vi "GetParam.vi"(8 "error in (no error)":errorcluster caption="entrée d'erreur (pas d'erreur)", 11 "Chi2_kernel.lvclass":refnum<class "Chi2_kernel.lvclass">) -> (0 "error out":errorcluster caption="sortie d'erreur", 2 "chi2_kernel":cluster{"gamma":dbl}={"gamma"=1.0}, 3 "Chi2_kernel.lvclass":refnum<class "Chi2_kernel.lvclass">)   [LabVIEW 2020, in "Chi2_kernel.lvclass"]
doc: "Get Parameters"
uses:
  Chi2_kernel.lvclass
  Chi2_kernel.lvclass/Chi2_kernel.ctl
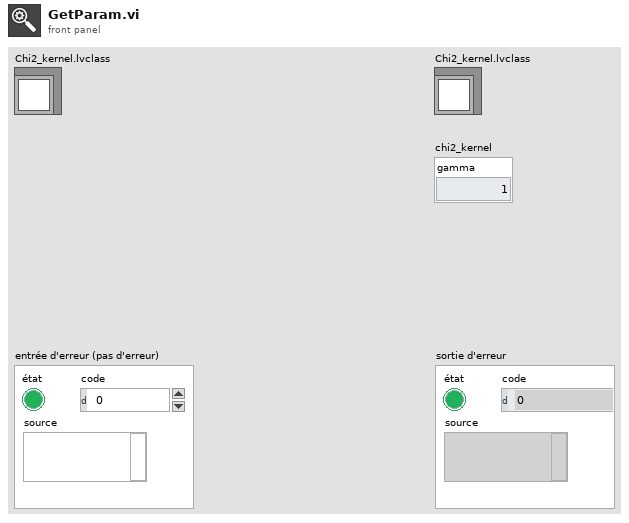
[diagram p1: front panel]
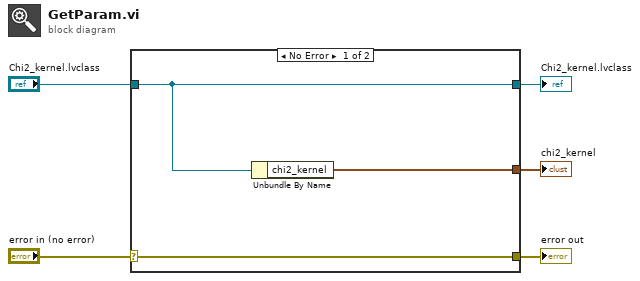
[diagram p0: block diagram]
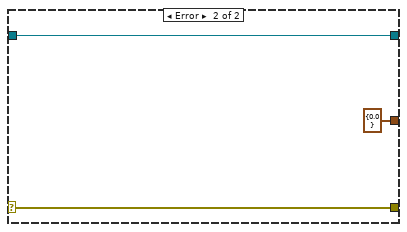
[diagram p2: hidden frame]
diagram:
  n1 = case shown="No Error" "error in (no error)" {
    selector: "error in (no error)" -> [w8 w10]
    tunnel: [w8 w10] -> w4
    tunnel: [w7 w11] -> w2
    tunnel: "Chi2_kernel.lvclass" -> [w7 w11]
    tunnel: [w6 cluster{"gamma":dbl} {"gamma"=0.0} ("chi2_kernel")] -> w1
    frame No Error {
      n2 = Unbundle By Name(w7) -> ("chi2_kernel"=w6:cluster{"gamma":dbl})
    }
    frame Error {
    }
  }
  "error out" <- w4
  "Chi2_kernel.lvclass" <- w2
  "chi2_kernel" <- w1
